vi "AR-DI-read.vi"(8 "error in":errorcluster, 11 "DI task in":refnum<k21>) -> (0 "error out":errorcluster, 2 "Data":bool[](array[boolean]), 3 "DI task out":refnum<k21>)   [LabVIEW 2021]
uses:
  <vilib>/DAQmx/read.llb/DAQmx Read (Digital 1D Bool 1Chan 1Samp).vi
  <vilib>/DAQmx/miscellaneous.llb/DAQmx Fill In Error Info.vi
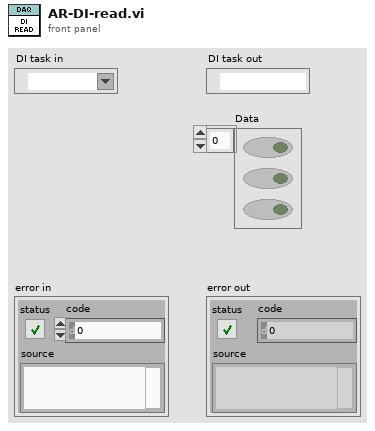
[diagram p1: front panel]
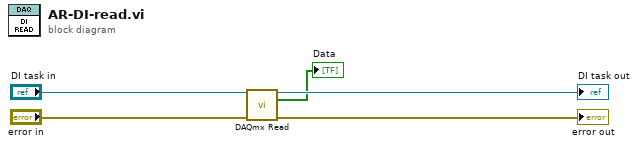
[diagram p0: block diagram]
diagram:
  n1 = call-poly <vilib>:"DAQmx Read.vi"("task/channels in"="DI task in", "error in"="error in") -> ("task out"=→"DI task out":refnum<k21>, "data"=→"Data":bool[], "error out"=→"error out":errorcluster)  [unwired: 11 in]
